vi "SignalWaveGen.vi"(4 "overScanBlanking":bool, 5 "Numeric 2":u16, 6 "numPts":i32, 7 "Numeric":u16, 9 "numRoundingPts":u16, 10 "singleDirScan":bool, 11 "scanWaveForm":T2) -> (2 "fastBlanking":T1={"startFwd"=0, "endFwd"=0, "startBwd"=0, "endBwd"=0, "disableBlanking"=FALSE, "useFineCounter"=TRUE}, 3 "Array":dbl[](array[numeric]))   [LabVIEW 2016]
uses:
  controls/ScanWaveform.ctl
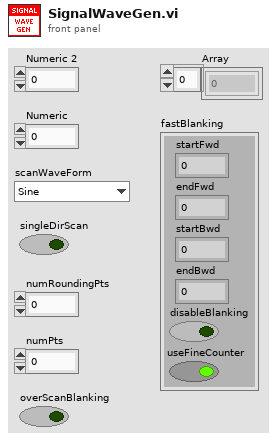
[diagram p1: front panel]
types:
  T1 = cluster{"startFwd":u16, "endFwd":u16, "startBwd":u16, "endBwd":u16, "disableBlanking":bool, "useFineCounter":bool}
  T2 = typedef "ScanWaveform.ctl" = enum16{"Sine", "Triangle", "Rounded"}
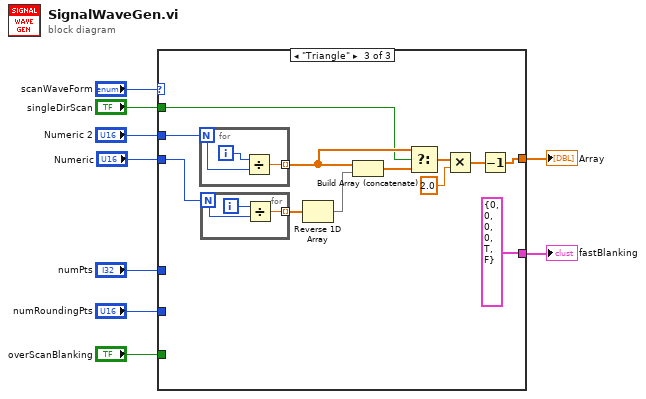
[diagram p0: block diagram]
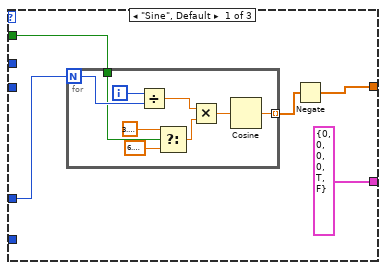
[diagram p2: hidden frame]
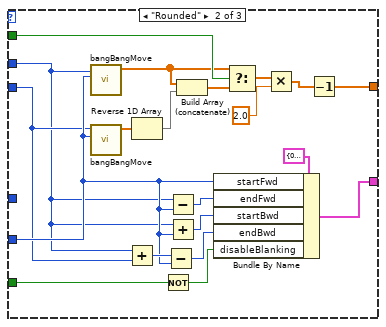
[diagram p3: hidden frame]
diagram:
  n1 = case shown="\"Triangle\"" "scanWaveForm" {
    tunnel: "singleDirScan" -> [w14 w38 w46]
    tunnel: "numRoundingPts" -> [_ w34 _]
    tunnel: [w11 w40 w45] -> w1
    tunnel: "overScanBlanking" -> [_ w32 _]
    tunnel: [T1 {"startFwd"=0, "endFwd"=0, "startBwd"=0, "endBwd"=0, "disableBlanking"=TRUE, "useFineCounter"=FALSE} ("fastBlanking") w30 T1 {"startFwd"=0, "endFwd"=0, "startBwd"=0, "endBwd"=0, "disableBlanking"=TRUE, "useFineCounter"=FALSE} ("fastBlanking")] -> w4
    tunnel: "Numeric 2" -> [_ w26 w55]
    tunnel: "Numeric" -> [_ w29 w54]
    tunnel: "numPts" -> [w12 _ _]
    frame "Sine", Default {
      n2 = for {
        N: w12 -> [w23]
        tunnel: w14 -> [w21]
        tunnel: [w15] -> w13 mode=indexing
        i -> [w22]
        n3 = Divide(x=w22, y=w23) -> (x/y=w17:dbl)
        n4 = Select(t=3.141592653589793, s=w21, f=6.283185307179586) -> (s? t:f=w18:dbl)
        n5 = Multiply(x=w17, y=w18) -> (x*y=w16:dbl)
        n6 = Cosine(x=w16) -> (cos(x)=w15:dbl)
      }
      n7 = Negate(x=w13) -> (-x=w11:dbl[])
    }
    frame "Rounded" {
      n8 = call "bangBangMove.vi"("numRoundingPts"=w34, "numPts"=w26) -> ("roundedHalfTriangle"=w28:dbl[])  [unwired: 9 in]
      n9 = call "bangBangMove.vi"("numRoundingPts"=w34, "numPts"=w29) -> ("roundedHalfTriangle"=w43:dbl[])  [unwired: 9 in]
      n10 = Add(x=w26, y=w29) -> (x+y=w35:u16)
      n11 = Reverse 1D Array(array=w43) -> (reversed array=w27:dbl[])
      n12 = Not(x=w32) -> (.not. x?=w31:bool)
      n13 = Subtract(x=w35, y=w34) -> (x-y=w33:u16)
      n14 = Subtract(x=w26, y=w34) -> (x-y=w37:u16)
      n15 = Add(x=w26, y=w34) -> (x+y=w36:u16)
      n16 = Build Array (concatenate)(w28, w27) -> (w42:dbl[])
      n17 = Bundle By Name(cluster=T1 {"startFwd"=0, "endFwd"=0, "startBwd"=0, "endBwd"=0, "disableBlanking"=FALSE, "useFineCounter"=FALSE} ("fastBlanking"), "startFwd"=w34, "endFwd"=w37, "startBwd"=w36, "endBwd"=w33, "disableBlanking"=w31) -> (w30:T1)
      n18 = Select(t=w28, s=w38, f=w42) -> (s? t:f=w39:dbl[])
      n19 = Multiply(x=w39, y=2.0) -> (x*y=w24:dbl[])
      n20 = Decrement(x=w24) -> (x-1=w40:dbl[])
    }
    frame "Triangle" {
      n21 = for {
        N: w55 -> [w60]
        tunnel: [w59] -> w47 mode=indexing
        i -> [w61]
        n22 = Divide(x=w61, y=w60) -> (x/y=w59:dbl)
      }
      n23 = for {
        N: w54 -> [w57]
        tunnel: [w56] -> w53 mode=indexing
        i -> [w58]
        n24 = Divide(x=w58, y=w57) -> (x/y=w56:dbl)
      }
      n25 = Reverse 1D Array(array=w53) -> (reversed array=w48:dbl[])
      n26 = Build Array (concatenate)(w47, w48) -> (w49:dbl[])
      n27 = Select(t=w47, s=w46, f=w49) -> (s? t:f=w52:dbl[])
      n28 = Multiply(x=w52, y=2.0) -> (x*y=w50:dbl[])
      n29 = Decrement(x=w50) -> (x-1=w45:dbl[])
    }
  }
  "fastBlanking" <- w4
  "Array" <- w1
